vi "Verify AND Combos.vi"(8 "error in":errorcluster) -> (0 "error in out":errorcluster)   [LabVIEW 2020, in "Caraya Extension Tests.lvclass"]
uses:
  Caraya Extension Tests.lvclass
  f0b51538-8a42-4750-ab89-e9f14ef91f99.vi
  Source/Extensions/Caraya.Extension/Caraya.Extension.lvlib
  <vilib>/addons/_JKI Toolkits/Caraya/classes/Test/Test.lvclass
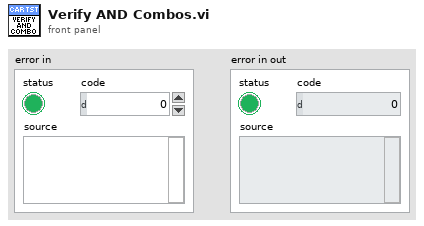
[diagram p1: front panel]
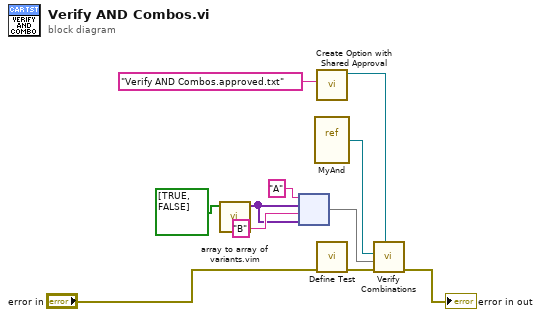
[diagram p0: block diagram]
diagram:
  n1 = call "array to array of variants.vim"("Array in"=bool[] [TRUE, FALSE]) -> ("Array out"=w5:variant[])  [unwired: 10 in]
  n2 = node ("Build Map")("A" ("key"), w5, "B" ("key"), w5) -> (w3:map{string, variant[]})
  n3 = vi-ref "MyAnd.vi"() -> (w4:refnum<vi>)
  n4 = call "Create Option with Shared Approval.vi"("Filename"="Verify AND Combos.approved.txt") -> ("Options outs"=w1:refnum<class "Options.lvclass">)  [unwired: 10 in]
  n5 = call <vilib>:"Define Test.vi"("error in (no error)"="error in") -> ("error out"=w11:errorcluster)  [unwired: 9 in, 1 out]
  n6 = call "Verify Combinations.vi"("Options"=w1, "error in"=w11, "ctl label -> value var[]"=w3, "VI Refnum"=w4) -> ("error out"=→"error in out":errorcluster)  [unwired: 6 in, 1 out]
